vi "Destructor.vi"(8 "error in (no error)":errorcluster, 11 "CollectionByRef in":refnum<class "CollectionByRef.lvclass">) -> (0 "error out":errorcluster)   [LabVIEW 2021, in "Collection.lvlib" / "CollectionByRef.lvclass"]
uses:
  CollectionByRef.lvclass
  CollectionByRef.lvclass/CollectionByRef.ctl
  CollectionByValue/CollectionByValue.lvclass
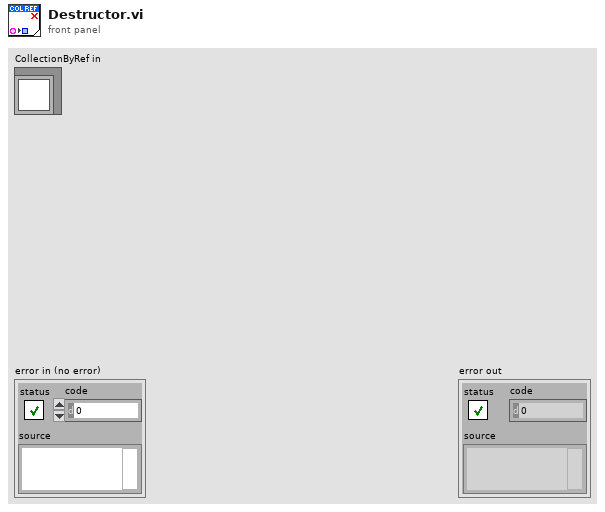
[diagram p1: front panel]
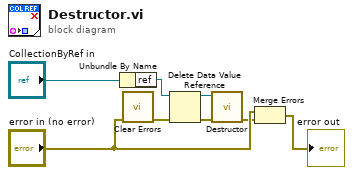
[diagram p0: block diagram]
diagram:
  n1 = Unbundle By Name("CollectionByRef in") -> ("ref"=w7:refnum<data-value>)
  n2 = call <vilib>:"Clear Errors.vi"("error in (no error)"="error in (no error)") -> ("error out"=w6:errorcluster)  [unwired: 5 in, 1 out]
  n3 = Delete Data Value Reference(data value reference=w7, error in=w6) -> (data value=w4:refnum<class "CollectionByValue.lvclass">, error out=w5:errorcluster)
  n4 = call "Destructor.vi"("error in (no error)"=w5, "Collection in"=w4) -> ("error out"=w2:errorcluster)  [unwired: 9 in]
  n5 = Merge Errors("error in (no error)", w2) -> (→"error out":errorcluster)
